vi "getPositions2string.vi"(10 "Moves":T1[](array[typedef])) -> (2 "Array":string[][](array[string]), 3 "spreadsheet string":string)   [LabVIEW 2019]
uses:
  APARMainSubvis/VXM Public API/singleAxisMoveDef.ctl
  APARMainSubvis/VXM Public API/mmWaveAxis.ctl
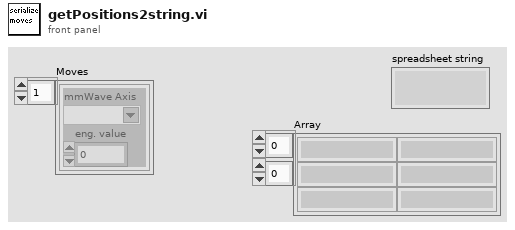
[diagram p1: front panel]
types:
  T1 = typedef "singleAxisMoveDef.ctl" = cluster{"mmWave Axis":T2, "eng. value":dbl}
  T2 = typedef "mmWaveAxis.ctl" = string
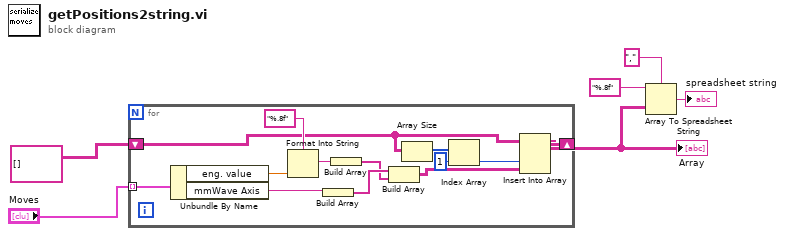
[diagram p0: block diagram]
diagram:
  n1 = for {
    tunnel: "Moves" -> [w19] mode=indexing
    shift-right: [w16] -> w3
    shift-left: string[][] [] -> [w12]
    n2 = Unbundle By Name(w19) -> ("eng. value"=w17:dbl, "mmWave Axis"=w15:T2)
    n3 = Format Into String(format string="%.8f", w17) -> (resulting string=w14:string)  [unwired: 2 in, 1 out]
    n4 = Build Array(w15) -> (w8:T2[])
    n5 = Build Array(w14) -> (w7:string[])
    n6 = Build Array(w8, w7) -> (w13:T2[][])
    n7 = Array Size(array=w12) -> (size(s)=w11:i32[])
    n8 = Index Array(array=w11, index=1) -> (element=w9:i32)
    n9 = Insert Into Array(array=w12, index (col)=w9, new element=w13) -> (w16:string[][])  [unwired: 1 in]
  }
  "Array" <- w3
  n10 = Array To Spreadsheet String(delimiter (Tab)=",", array=w3, 3:"%.8f" ("format string")) -> (spreadsheet string=→"spreadsheet string":string)
